vi "IT8511Control.vi"(0 "Port":string="ª\u0001&\u0000'", 1 "baud rate (9600)":u32=9600 caption="波特率(9600)", 2 "function":T1(ring), 3 "volt set (V)":u32, 4 "curr set (MA)":dbl) -> (20 "volt out":dbl, 21 "curr out":dbl, 22 "result":i32=2)   [LabVIEW 2018]
uses:
  <vilib>/Instr/_visa.llb/VISA Configure Serial Port (Instr).vi
panel:
  out "error out":errorcluster
  # "IT8511Control"
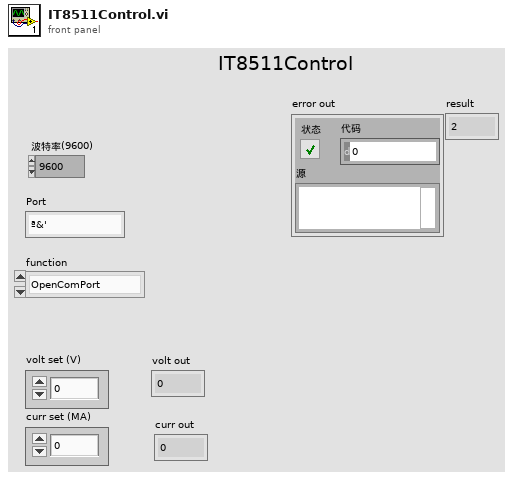
[diagram p1: front panel]
types:
  T1 = enum16{"OpenComPort", "SetCurrent", "ReadVoltAndCurrent", "OutPut ON", "OutPUt OFF", "RemoteMode", "LocalMode", "CCMode", "CVMode", "CloseComPort"}
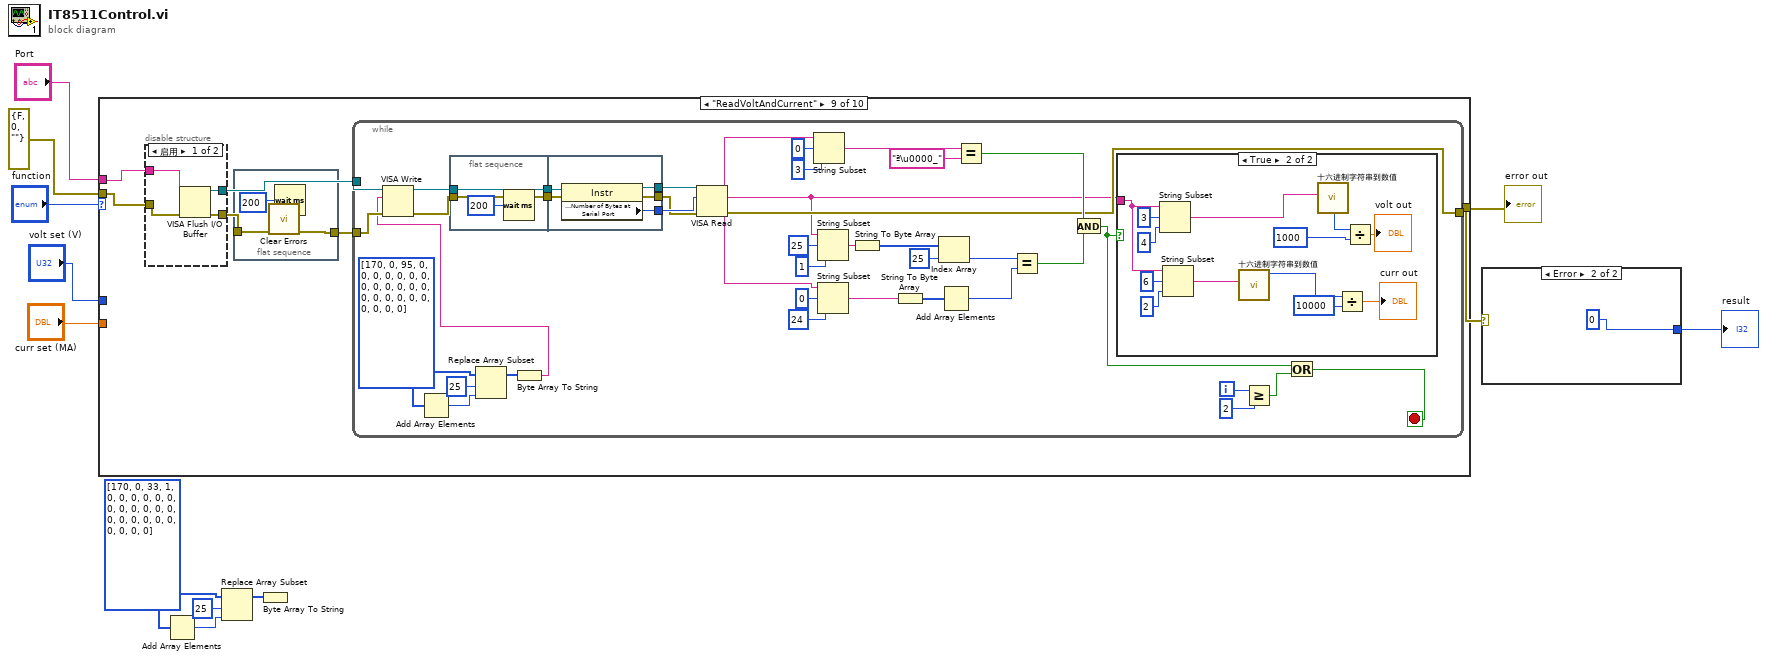
[diagram p0: block diagram]
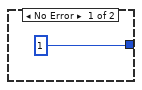
[diagram p2: hidden frame]
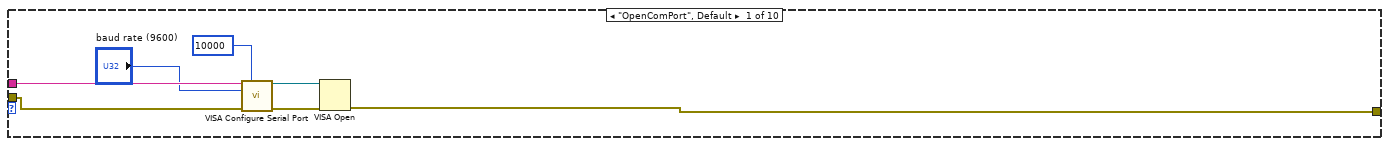
[diagram p3: hidden frame]
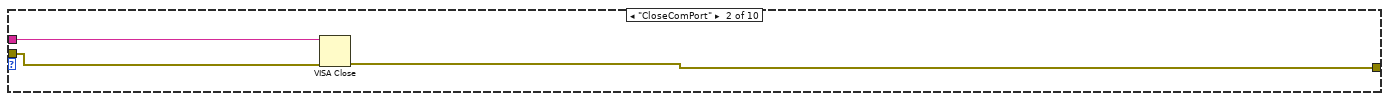
[diagram p4: hidden frame]
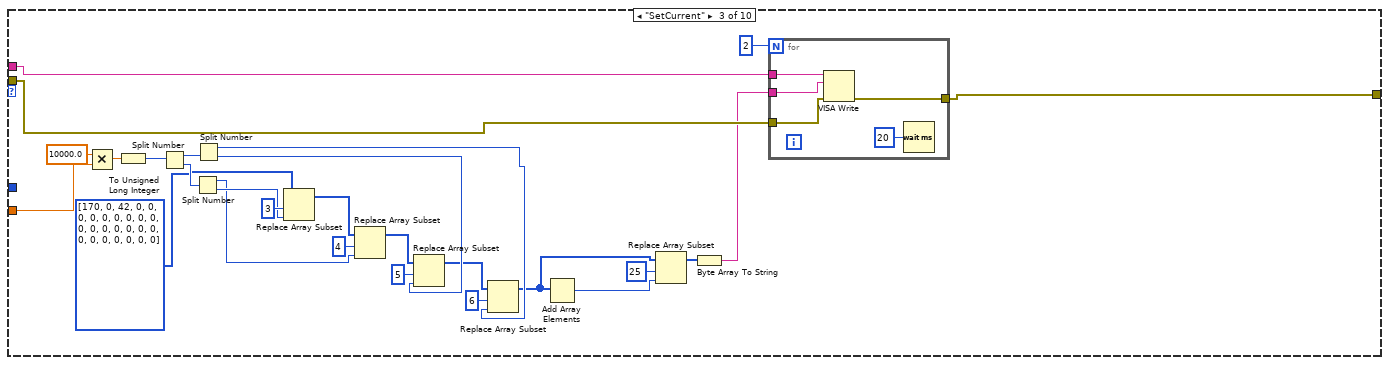
[diagram p5: hidden frame]
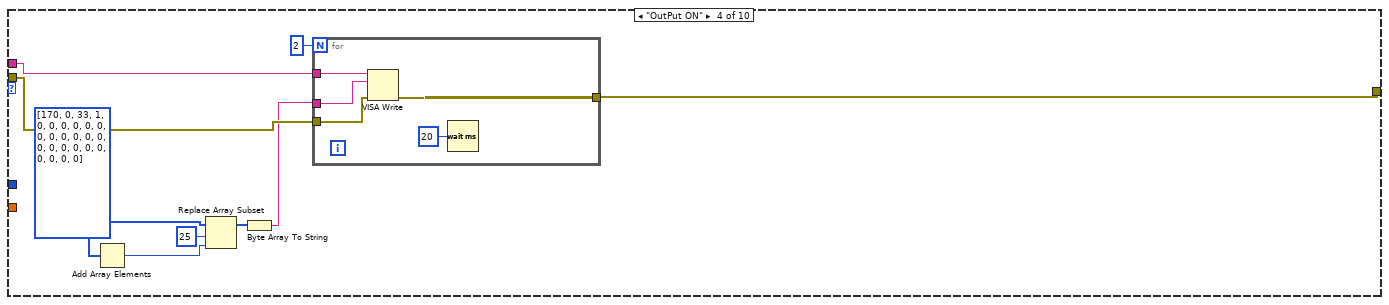
[diagram p6: hidden frame]
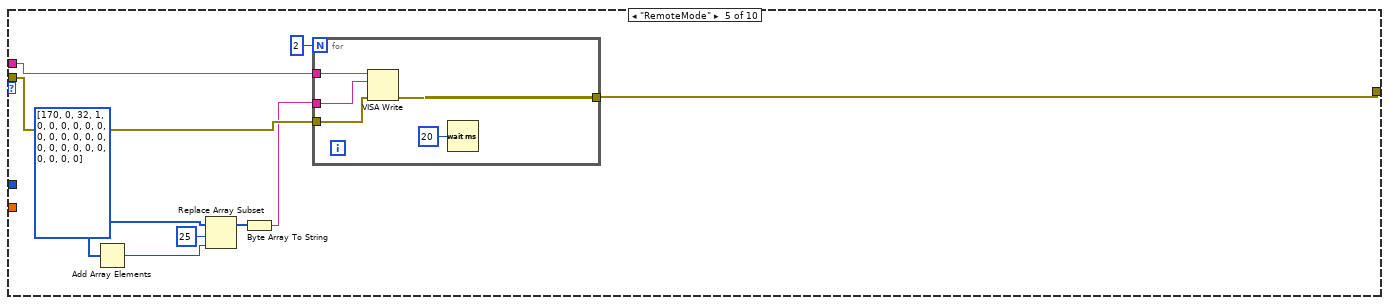
[diagram p7: hidden frame]
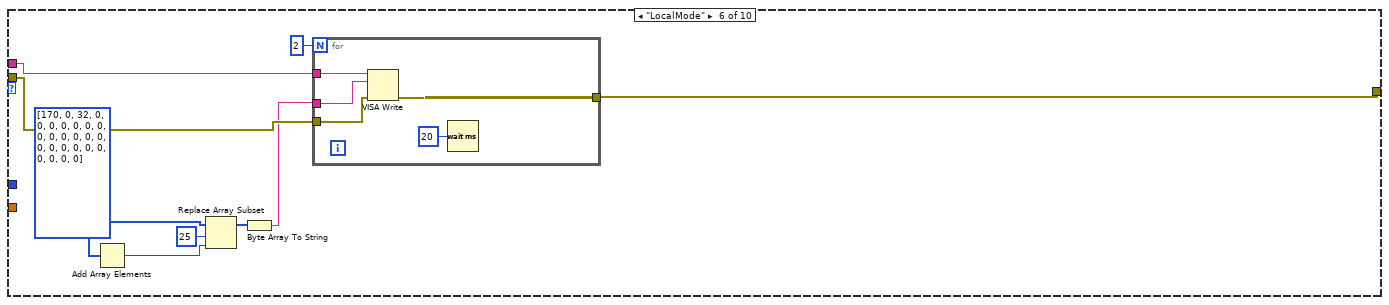
[diagram p8: hidden frame]
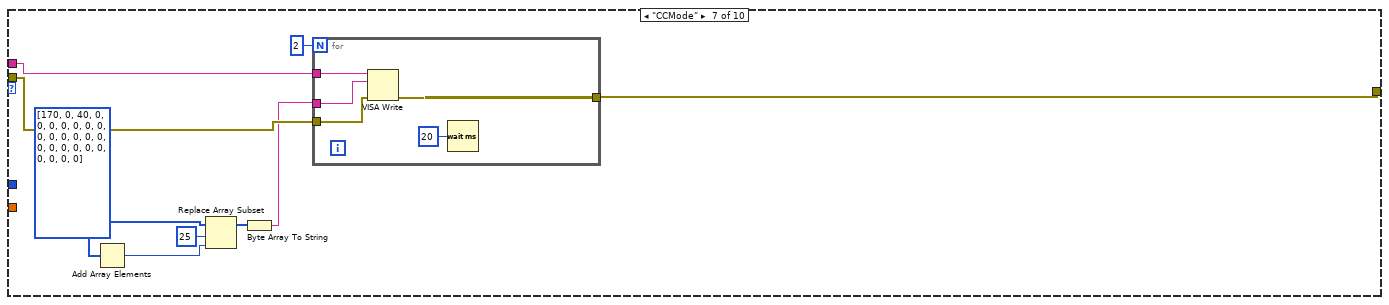
[diagram p9: hidden frame]
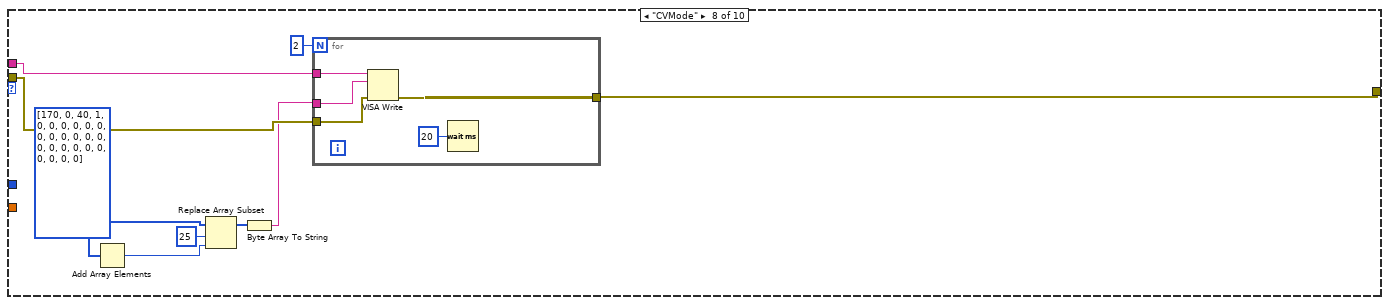
[diagram p10: hidden frame]
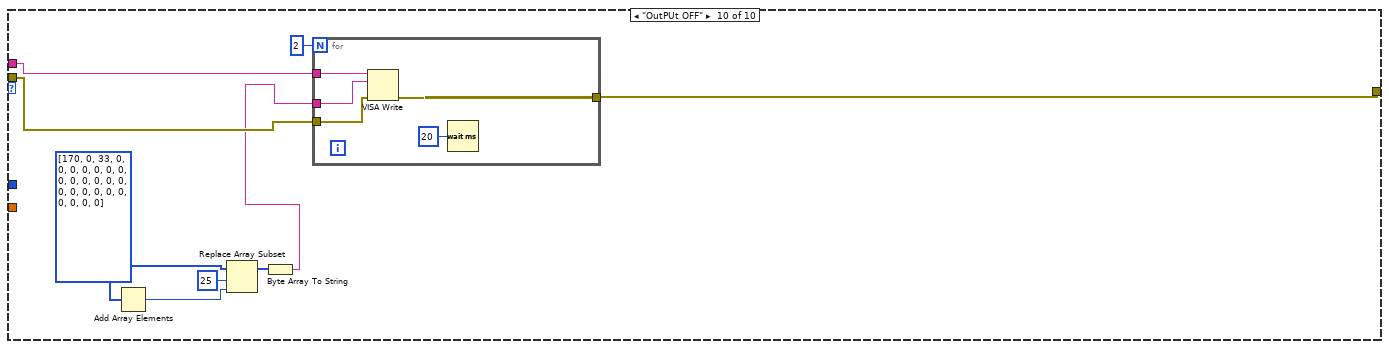
[diagram p13: hidden frame]
diagram:
  w2 = u8[] [170, 0, 33, 1, 0, 0, 0, 0, 0, 0, 0, 0, 0, 0, 0, 0, 0, 0, 0, 0, 0, 0, 0, 0, 0, 0]
  n1 = case shown="\"ReadVoltAndCurrent\"" "function" {
    tunnel: "Port" -> [w16 w20 w47 w61 w75 w89 w103 w117 w127 w205]
    tunnel: errorcluster {"status"=FALSE, "code"=0, "source"=""} ("error in (no error)") -> [w15 w19 w46 w60 w74 w88 w102 w116 w126 w204]
    tunnel: [w14 w21 w45 w59 w73 w87 w101 w115 w129 w203] -> w6
    tunnel: "curr set (MA)" -> [_ _ w42 _ _ _ _ _ _ _]
    tunnel: "volt set (V)" -> [_ _ _ _ _ _ _ _ _ _]
    frame "OpenComPort", Default {
      n2 = call-poly "VISA Configure Serial Port"("VISA resource name"=w16, "timeout (10sec)"=u32 10000, "baud rate (9600)"="baud rate (9600)", "error in (no error)"=w15) -> ("VISA resource name out"=w18:refnum<visa-resource-name>, "error out"=w17:errorcluster)  [unwired: 10 in]
      n3 = VISA Open(error in (no error)=w17, VISA resource name=w18) -> (error out=w14:errorcluster)  [unwired: 3 in, 1 out]
    }
    frame "CloseComPort" {
      n4 = VISA Close(VISA resource name=w20, error in (no error)=w19) -> (error out=w21:errorcluster)
    }
    frame "SetCurrent" {
      n5 = Multiply(x=10000.0, y=w42) -> (x*y=w44:dbl)
      n6 = To Unsigned Long Integer(number=w44) -> (unsigned 32bit integer=w38:u32)
      n7 = Split Number(x=w38) -> (hi(x)=w37:u16, lo(x)=w36:u16)
      n8 = Split Number(x=w36) -> (hi(x)=w30:u8, lo(x)=w31:u8)
      n9 = Split Number(x=w37) -> (hi(x)=w24:u8, lo(x)=w26:u8)
      n10 = Replace Array Subset(array=u8[] [170, 0, 42, 0, 0, 0, 0, 0, 0, 0, 0, 0, 0, 0, 0, 0, 0, 0, 0, 0, 0, 0, 0, 0, 0, 0], new element=w31, index=3) -> (w32:u8[])
      n11 = Replace Array Subset(array=w32, new element=w30, index=4) -> (w27:u8[])
      n12 = Replace Array Subset(array=w27, new element=w26, index=5) -> (w25:u8[])
      n13 = Replace Array Subset(array=w25, new element=w24, index=6) -> (w23:u8[])
      n14 = Add Array Elements(numeric array=w23) -> (sum=w40:u8)
      n15 = Replace Array Subset(array=w23, new element=w40, index=25) -> (w39:u8[])
      n16 = Byte Array To String(unsigned byte array=w39) -> (string=w22:string)
      n17 = for {
        N: 2 -> [_]
        tunnel: [w53] -> w45
        tunnel: w47 -> [w52]
        tunnel: w46 -> [w51]
        tunnel: w22 -> [w49]
        n18 = VISA Write(VISA resource name=w52, write buffer=w49, error in (no error)=w51) -> (error out=w53:errorcluster)  [unwired: 2 out]
        n19 = Wait (ms)(milliseconds to wait=u32 20 ("等待时间（毫秒）")) -> ()  [unwired: 1 out]
      }
    }
    frame "OutPut ON" {
      w58 = u8[] [170, 0, 33, 1, 0, 0, 0, 0, 0, 0, 0, 0, 0, 0, 0, 0, 0, 0, 0, 0, 0, 0, 0, 0, 0, 0]
      n20 = Add Array Elements(numeric array=w58) -> (sum=w56:u8)
      n21 = Replace Array Subset(array=w58, new element=w56, index=25) -> (w55:u8[])
      n22 = Byte Array To String(unsigned byte array=w55) -> (string=w54:string)
      n23 = for {
        N: 2 -> [_]
        tunnel: [w67] -> w59
        tunnel: w61 -> [w66]
        tunnel: w54 -> [w65]
        tunnel: w60 -> [w64]
        n24 = VISA Write(VISA resource name=w66, write buffer=w65, error in (no error)=w64) -> (error out=w67:errorcluster)  [unwired: 2 out]
        n25 = Wait (ms)(milliseconds to wait=u32 20 ("等待时间（毫秒）")) -> ()  [unwired: 1 out]
      }
    }
    frame "RemoteMode" {
      w72 = u8[] [170, 0, 32, 1, 0, 0, 0, 0, 0, 0, 0, 0, 0, 0, 0, 0, 0, 0, 0, 0, 0, 0, 0, 0, 0, 0]
      n26 = Add Array Elements(numeric array=w72) -> (sum=w70:u8)
      n27 = Replace Array Subset(array=w72, new element=w70, index=25) -> (w69:u8[])
      n28 = Byte Array To String(unsigned byte array=w69) -> (string=w68:string)
      n29 = for {
        N: 2 -> [_]
        tunnel: [w81] -> w73
        tunnel: w75 -> [w80]
        tunnel: w68 -> [w79]
        tunnel: w74 -> [w78]
        n30 = VISA Write(VISA resource name=w80, write buffer=w79, error in (no error)=w78) -> (error out=w81:errorcluster)  [unwired: 2 out]
        n31 = Wait (ms)(milliseconds to wait=u32 20 ("等待时间（毫秒）")) -> ()  [unwired: 1 out]
      }
    }
    frame "LocalMode" {
      w86 = u8[] [170, 0, 32, 0, 0, 0, 0, 0, 0, 0, 0, 0, 0, 0, 0, 0, 0, 0, 0, 0, 0, 0, 0, 0, 0, 0]
      n32 = Add Array Elements(numeric array=w86) -> (sum=w84:u8)
      n33 = Replace Array Subset(array=w86, new element=w84, index=25) -> (w83:u8[])
      n34 = Byte Array To String(unsigned byte array=w83) -> (string=w82:string)
      n35 = for {
        N: 2 -> [_]
        tunnel: [w95] -> w87
        tunnel: w89 -> [w94]
        tunnel: w82 -> [w93]
        tunnel: w88 -> [w92]
        n36 = VISA Write(VISA resource name=w94, write buffer=w93, error in (no error)=w92) -> (error out=w95:errorcluster)  [unwired: 2 out]
        n37 = Wait (ms)(milliseconds to wait=u32 20 ("等待时间（毫秒）")) -> ()  [unwired: 1 out]
      }
    }
    frame "CCMode" {
      w100 = u8[] [170, 0, 40, 0, 0, 0, 0, 0, 0, 0, 0, 0, 0, 0, 0, 0, 0, 0, 0, 0, 0, 0, 0, 0, 0, 0]
      n38 = Add Array Elements(numeric array=w100) -> (sum=w98:u8)
      n39 = Replace Array Subset(array=w100, new element=w98, index=25) -> (w97:u8[])
      n40 = Byte Array To String(unsigned byte array=w97) -> (string=w96:string)
      n41 = for {
        N: 2 -> [_]
        tunnel: [w109] -> w101
        tunnel: w103 -> [w108]
        tunnel: w96 -> [w107]
        tunnel: w102 -> [w106]
        n42 = VISA Write(VISA resource name=w108, write buffer=w107, error in (no error)=w106) -> (error out=w109:errorcluster)  [unwired: 2 out]
        n43 = Wait (ms)(milliseconds to wait=u32 20 ("等待时间（毫秒）")) -> ()  [unwired: 1 out]
      }
    }
    frame "CVMode" {
      w114 = u8[] [170, 0, 40, 1, 0, 0, 0, 0, 0, 0, 0, 0, 0, 0, 0, 0, 0, 0, 0, 0, 0, 0, 0, 0, 0, 0]
      n44 = Add Array Elements(numeric array=w114) -> (sum=w112:u8)
      n45 = Replace Array Subset(array=w114, new element=w112, index=25) -> (w111:u8[])
      n46 = Byte Array To String(unsigned byte array=w111) -> (string=w110:string)
      n47 = for {
        N: 2 -> [_]
        tunnel: [w123] -> w115
        tunnel: w117 -> [w122]
        tunnel: w110 -> [w121]
        tunnel: w116 -> [w120]
        n48 = VISA Write(VISA resource name=w122, write buffer=w121, error in (no error)=w120) -> (error out=w123:errorcluster)  [unwired: 2 out]
        n49 = Wait (ms)(milliseconds to wait=u32 20 ("等待时间（毫秒）")) -> ()  [unwired: 1 out]
      }
    }
    frame "ReadVoltAndCurrent" {
      n50 = disable-structure shown="启用" {
        disable-tunnel: w127 -> [w133 w135]
        disable-tunnel: w126 -> [w132 w134]
        disable-tunnel: [w131 w135] -> w125
        disable-tunnel: [w130 w134] -> w124
        frame Enabled {
          n51 = VISA Flush I/O Buffer(VISA resource name=w133, error in (no error)=w132) -> (VISA resource name out=w131:refnum<visa-resource-name>, error out=w130:errorcluster)  [unwired: 1 in]
        }
        frame Disabled {
        }
      }
      n52 = flat-sequence {
        tunnel: [w138] -> w128
        tunnel: w124 -> [w137]
        frame #0 {
          n53 = call <vilib>:"Clear Errors.vi"("error in (no error)"=w137) -> ("error out"=w138:errorcluster)  [unwired: 5 in, 1 out]
          n54 = Wait (ms)(milliseconds to wait=u32 200 ("等待时间（毫秒）")) -> ()  [unwired: 1 out]
        }
      }
      n55 = while {
        tunnel: [w162] -> w129
        tunnel: w125 -> [w176]
        tunnel: w128 -> [w163]
        i -> [w165]
        stop <- w157 stop-if-true
        w154 = u8[] [170, 0, 95, 0, 0, 0, 0, 0, 0, 0, 0, 0, 0, 0, 0, 0, 0, 0, 0, 0, 0, 0, 0, 0, 0, 0]
        n56 = Add Array Elements(numeric array=w154) -> (sum=w153:u8)
        n57 = flat-sequence {
          tunnel: w166 -> [w178]
          tunnel: w174 -> [w179]
          tunnel: [w179] -> w161
          tunnel: [w178] -> w160
          tunnel: [w184] -> w175
          tunnel: [w182] -> w167
          tunnel: [w180] -> w156
          tunnel: w161 -> [w183]
          tunnel: w160 -> [w181]
          frame #0 {
            n58 = Wait (ms)(milliseconds to wait=u32 200 ("等待时间（毫秒）")) -> ()  [unwired: 1 out]
          }
          frame #1 {
            n59 = property class="Instr"(reference=w183, error in=w181) -> (reference out=w182:refnum<visa-resource-name>, error out=w180:errorcluster, "Serial Settings:Number of Bytes at Serial Port"=w184:u32)
          }
        }
        n60 = Replace Array Subset(array=w154, new element=w153, index=25) -> (w152:u8[])
        n61 = Byte Array To String(unsigned byte array=w152) -> (string=w151:string)
        n62 = VISA Write(VISA resource name=w176, write buffer=w151, error in (no error)=w163) -> (VISA resource name out=w174:refnum<visa-resource-name>, error out=w166:errorcluster)  [unwired: 1 out]
        n63 = VISA Read(VISA resource name=w167, byte count=w175, error in (no error)=w156) -> (read buffer=w141:string, error out=w162:errorcluster)  [unwired: 2 out]
        n64 = String Subset(string=w141, offset (0)=0 ("偏移量(0)"), length (rest)=3 ("长度（剩余）")) -> (substring=w140:string)
        n65 = String Subset(string=w141, offset (0)=25 ("偏移量(0)"), length (rest)=1 ("长度（剩余）")) -> (substring=w147:string)
        n66 = String Subset(string=w141, offset (0)=0 ("偏移量(0)"), length (rest)=24 ("长度（剩余）")) -> (substring=w149:string)
        n67 = String To Byte Array(string=w147) -> (unsigned byte array=w146:u8[])
        n68 = String To Byte Array(string=w149) -> (unsigned byte array=w150:u8[])
        n69 = Index Array(array=w146, index=25) -> (element=w145:u8)
        n70 = Add Array Elements(numeric array=w150) -> (sum=w148:u8)
        n71 = Equal?(x=w140, y="ª\u0000_") -> (x = y?=w169:bool)
        n72 = Equal?(x=w145, y=w148) -> (x = y?=w168:bool)
        n73 = And(x=w169, y=w168) -> (x .and. y?=w159:bool)
        n74 = case shown="True" w159 {
          tunnel: w141 -> [_ w187]
          frame False {
          }
          frame True {
            n75 = String Subset(string=w187, offset (0)=3 ("偏移量(0)"), length (rest)=4 ("长度（剩余）")) -> (substring=w186:string)
            n76 = String Subset(string=w187, offset (0)=6 ("偏移量(0)"), length (rest)=2 ("长度（剩余）")) -> (substring=w185:string)
            n77 = call "十六进制字符串到数值.vi"("字符串"=w185) -> ("数值"=w190:i32)  [unwired: 9 in, 1 out]
            n78 = call "十六进制字符串到数值.vi"("字符串"=w186) -> ("数值"=w195:i32)  [unwired: 9 in, 1 out]
            n79 = Divide(x=w190, y=10000) -> (x/y=→"curr out":dbl)
            n80 = Divide(x=w195, y=1000) -> (x/y=→"volt out":dbl)
          }
        }
        n81 = Greater Or Equal?(x=w165, y=2) -> (x >= y?=w158:bool)
        n82 = Or(x=w159, y=w158) -> (x .or. y?=w157:bool)
      }
    }
    frame "OutPUt OFF" {
      w202 = u8[] [170, 0, 33, 0, 0, 0, 0, 0, 0, 0, 0, 0, 0, 0, 0, 0, 0, 0, 0, 0, 0, 0, 0, 0, 0, 0]
      n83 = Add Array Elements(numeric array=w202) -> (sum=w200:u8)
      n84 = Replace Array Subset(array=w202, new element=w200, index=25) -> (w199:u8[])
      n85 = Byte Array To String(unsigned byte array=w199) -> (string=w198:string)
      n86 = for {
        N: 2 -> [_]
        tunnel: [w211] -> w203
        tunnel: w205 -> [w210]
        tunnel: w198 -> [w209]
        tunnel: w204 -> [w208]
        n87 = VISA Write(VISA resource name=w210, write buffer=w209, error in (no error)=w208) -> (error out=w211:errorcluster)  [unwired: 2 out]
        n88 = Wait (ms)(milliseconds to wait=u32 20 ("等待时间（毫秒）")) -> ()  [unwired: 1 out]
      }
    }
  }
  "error out" <- w6
  n89 = Add Array Elements(numeric array=w2) -> (sum=w3:u8)
  n90 = Replace Array Subset(array=w2, new element=w3, index=25) -> (w4:u8[])
  n91 = Byte Array To String(unsigned byte array=w4) -> ()  [unwired: 1 out]
  n92 = case shown="Error" w6 {
    tunnel: [1 ("y") 0 ("y")] -> w5
    frame No Error {
    }
    frame Error {
    }
  }
  "result" <- w5
